vi "Set_data_to_visual_UP.vi"(8 "error in (no error)":errorcluster, 11 "RFID system in":refnum<class "RFID system.lvclass">) -> (0 "error out":errorcluster, 2 "Visual":T1, 3 "RFID system out":refnum<class "RFID system.lvclass">)   [LabVIEW 2019]
uses:
  RFID system.lvclass
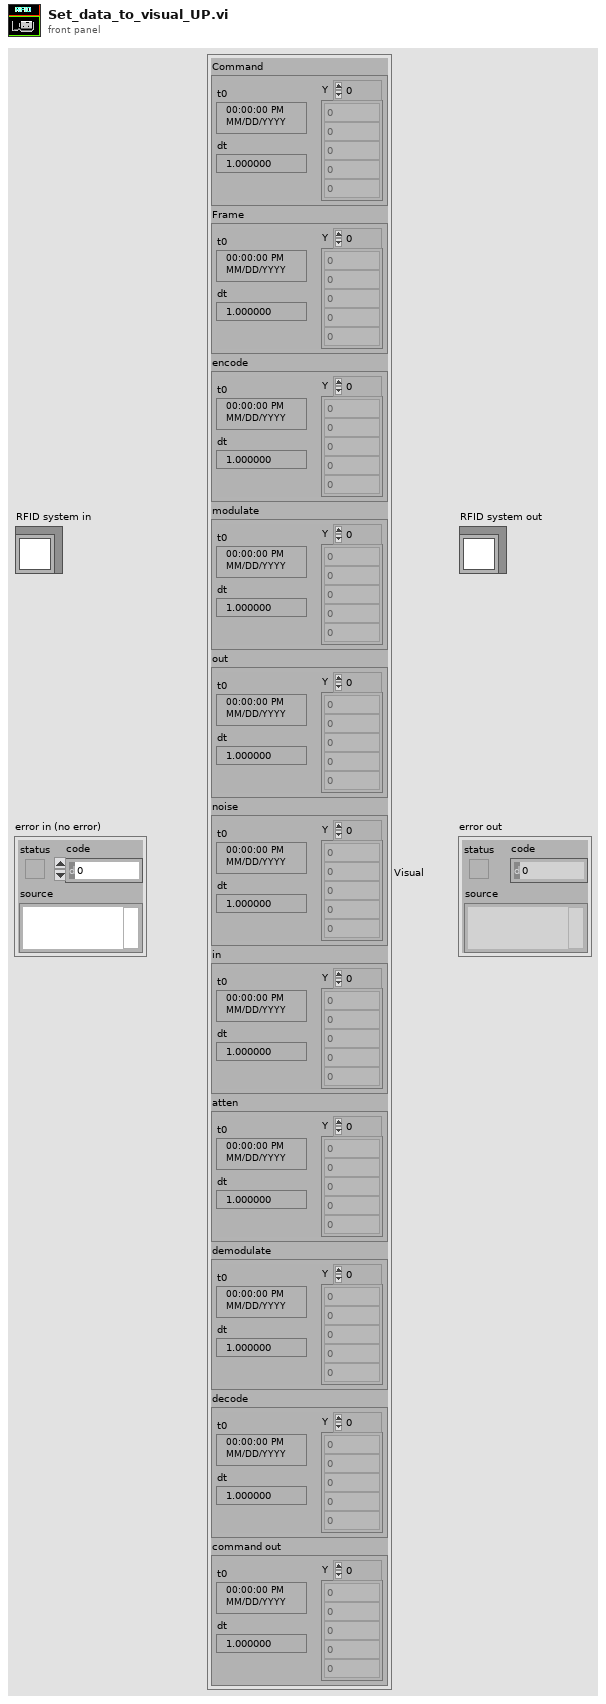
[diagram p1: front panel]
types:
  T1 = cluster{"Command":waveform(cdb), "Frame":waveform(cdb), "encode":waveform(cdb), "modulate":waveform(cdb), "out":waveform(cdb), "noise":waveform(cdb), "in":waveform(cdb), "atten":waveform(cdb), "demodulate":waveform(cdb), "decode":waveform(cdb), "command out":waveform(cdb)}
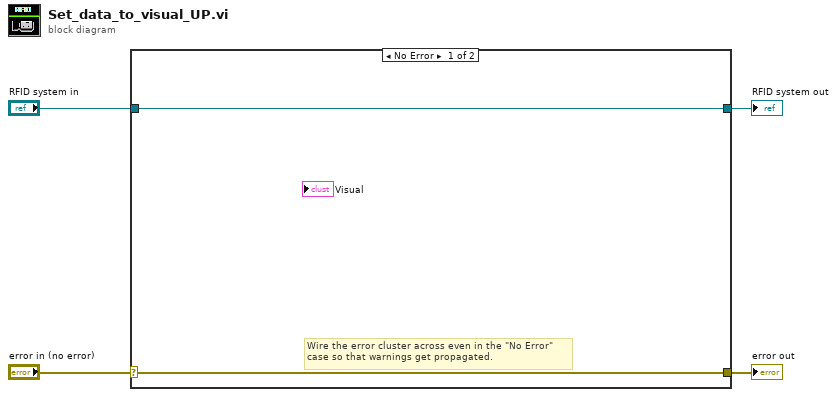
[diagram p0: block diagram]
diagram:
  n1 = case shown="No Error" "error in (no error)" {
    selector: "error in (no error)" -> [w5 w8]
    tunnel: [w5 w8] -> w3
    tunnel: [w6 w7] -> w1
    tunnel: "RFID system in" -> [w6 w7]
    frame No Error {
      # "Wire the error cluster across even in the \"No Error\"\ncase so that warnings get propagated."
    }
    frame Error {
    }
  }
  "error out" <- w3
  "RFID system out" <- w1
